vi "11 - Workspace discovery.vi"() -> ()   [LabVIEW 2020]
uses:
  client/client.lvlib
panel:
  out "Workspaces":string[](array[string])
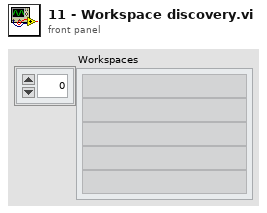
[diagram p1: front panel]
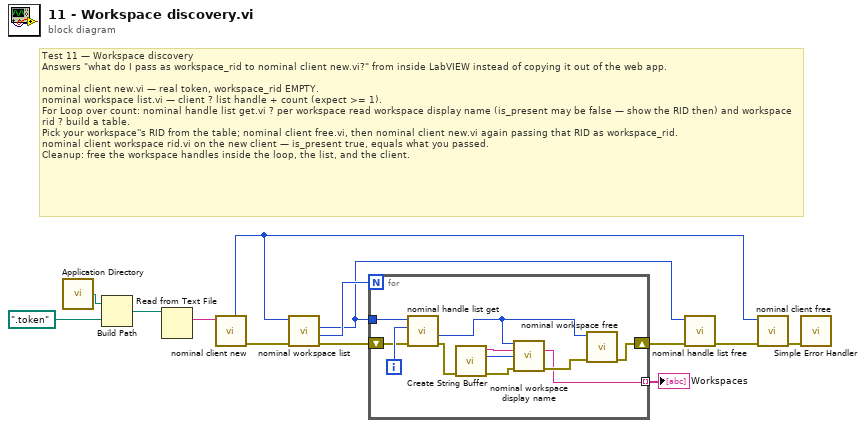
[diagram p0: block diagram]
diagram:
  # "Test 11 — Workspace discovery\nAnswers \"what do I pass as workspace_rid to nominal client new.vi?\" from inside LabVIEW instead of copying it out of the web app.\n\nnominal client new.vi — real token, workspace_rid EMPTY.\nnominal workspace list.vi — client ? list handle + count (expect >= 1).\nFor Loop over count: nominal handle list get.vi ? per workspace read workspace display name (is_present may be false — show the RID then) and workspace rid ? build a table.\nPick your workspace''s RID from the table; nominal client free.vi, then nominal client new.vi again passing that RID as workspace_rid.\nnominal client workspace rid.vi on the new client — is_present true, equals what you passed.\nCleanup: free the workspace handles inside the loop, the list, and the client."
  n1 = call <vilib>:"Application Directory.vi"() -> ("Application Directory"=w12:path)
  n2 = Build Path(base path=w12, name or relative path=path ".token") -> (appended path=w10:path)
  n3 = Read from Text File(file (use dialog)=w10) -> (text=w9:string)  [unwired: 3 in, 3 out]
  n4 = call "nominal client new.vi"("token"=w9) -> ("error out"=w8:errorcluster, "out_client out"=w3:i32)  [unwired: 8 in, 1 out]
  n5 = call "nominal workspace list.vi"("error in (no error)"=w8, "client"=w3) -> ("error out"=w6:errorcluster, "out_count out"=w7:u32, "out_list out"=w5:i32)  [unwired: 6 in, 1 out]
  n6 = for {
    N: w7 -> [_]
    tunnel: w5 -> [w24]
    shift-right: [w20] -> w4
    shift-left: w6 -> [w22]
    tunnel: [w14] -> w1 mode=indexing
    i -> [w23]
    n7 = call "nominal handle list get.vi"("error in (no error)"=w22, "index"=w23, "list"=w24) -> ("error out"=w21:errorcluster, "out_handle out"=w19:i32)  [unwired: 6 in, 1 out]
    n8 = call "Create String Buffer.vi"("error in"=w21) -> ("error out"=w15:errorcluster, "dub Buffer Size"=w17:i32, "String Buffer"=w18:string)  [unwired: 8 in]
    n9 = call "nominal workspace display name.vi"("workspace"=w19, "buf"=w18, "cap"=w17, "error in (no error)"=w15) -> ("buf out"=w14:string, "error out"=w16:errorcluster)  [unwired: 7 in, 3 out]
    n10 = call "nominal workspace free.vi"("error in (no error)"=w16, "workspace"=w19) -> ("error out"=w20:errorcluster)  [unwired: 8 in, 1 out]
  }
  "Workspaces" <- w1
  n11 = call "nominal handle list free.vi"("error in (no error)"=w4, "list"=w5) -> ("error out"=w2:errorcluster)  [unwired: 8 in, 1 out]
  n12 = call "nominal client free.vi"("error in (no error)"=w2, "client"=w3) -> ("error out"=w13:errorcluster)  [unwired: 8 in, 1 out]
  n13 = call <vilib>:"Simple Error Handler.vi"("error in (no error)"=w13) -> ()  [unwired: 4 in, 5 out]
